vi "Write Connection Configuration.vi"(8 "error in (no error)":errorcluster, 10 "Connection Configuration":T1, 11 "SystemLink configuration in":refnum<class "SystemLink configuration.lvclass">) -> (0 "error out":errorcluster, 3 "SystemLink configuration out":refnum<class "SystemLink configuration.lvclass">)   [LabVIEW 2015, in "SystemLink configuration.lvclass"]
uses:
  SystemLink configuration.lvclass
  Connection Configuration.ctl
  Connection Type.ctl
  SystemLink configuration.lvclass/SystemLink configuration.ctl
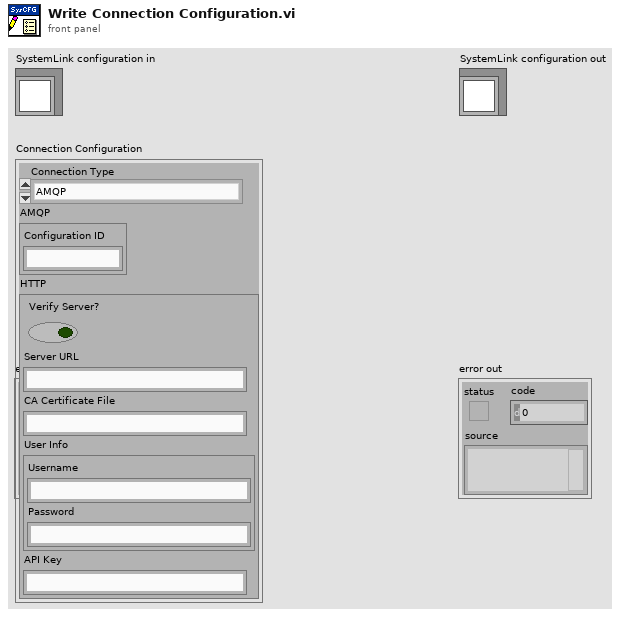
[diagram p1: front panel]
types:
  T1 = typedef "SystemLink configuration.lvclass/Connection Configuration.ctl" = cluster{"Connection Type":T2, "AMQP":cluster{"Configuration ID":string}, "HTTP":cluster{"Verify Server?":bool, "Server URL":string, "CA Certificate File":string, "User Info":cluster{"Username":string, "Password":string}, "API Key":string}}
  T2 = typedef "SystemLink configuration.lvclass/Connection Type.ctl" = enum16{"AMQP", "HTTP", "API Key (SystemLink Cloud)"}
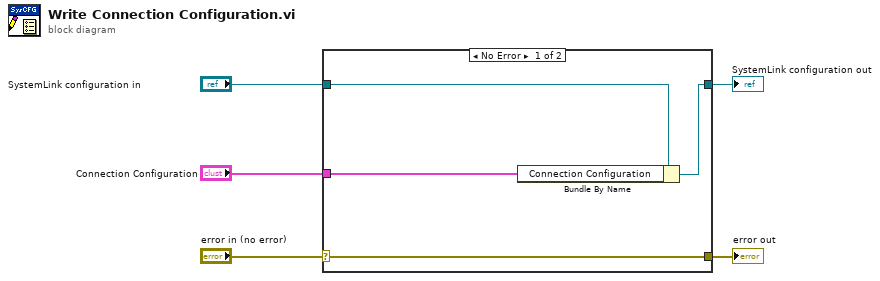
[diagram p0: block diagram]
diagram:
  n1 = case shown="No Error" "error in (no error)" {
    selector: "error in (no error)" -> [w9 w10]
    tunnel: [w9 w10] -> w4
    tunnel: [w7 w11] -> w2
    tunnel: "SystemLink configuration in" -> [w8 w11]
    tunnel: "Connection Configuration" -> [w6 _]
    frame No Error {
      n2 = Bundle By Name(cluster=w8, "Connection Configuration"=w6) -> (w7:refnum<class "SystemLink configuration.lvclass">)
    }
    frame Error {
    }
  }
  "error out" <- w4
  "SystemLink configuration out" <- w2
